vi "locate tag.vi"(8 "error in":errorcluster, 10 "name":string, 11 "data dictionary in":refnum<class "data bus dictionary.lvclass">) -> (0 "error out":errorcluster, 1 "data type":T1, 2 "index":i32, 3 "data dictionary out":refnum<class "data bus dictionary.lvclass">)   [LabVIEW 2013, in "data bus dictionary.lvclass"]
doc: "Locates a tag in the data dictionary and returns its index within the data table."
uses:
  data bus dictionary.lvclass
  tag/Data Type.ctl
  data bus dictionary.lvclass/data bus dictionary.ctl
  dictionary lookup value.ctl
  tag/data bus tag description.lvclass
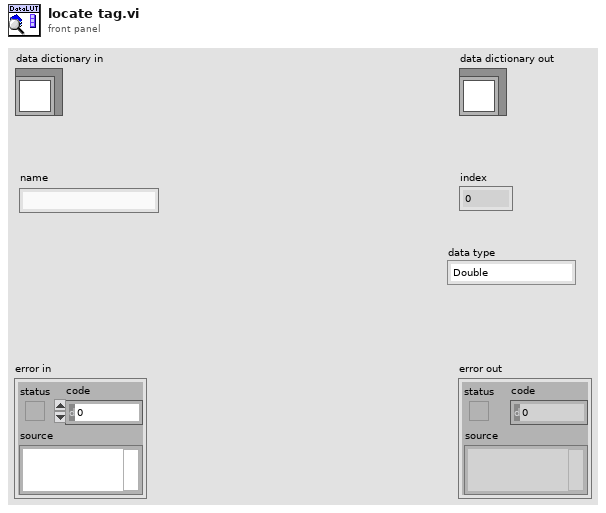
[diagram p1: front panel]
types:
  T1 = typedef "data bus tag description.lvclass/Data Type.ctl" = enum16{"Double", "I64", "Boolean", "Array of Double", "Array of I64", "Variant"}
  T2 = typedef "data bus dictionary.lvclass/dictionary lookup value.ctl" = cluster{"data type":T1, "index":i32}
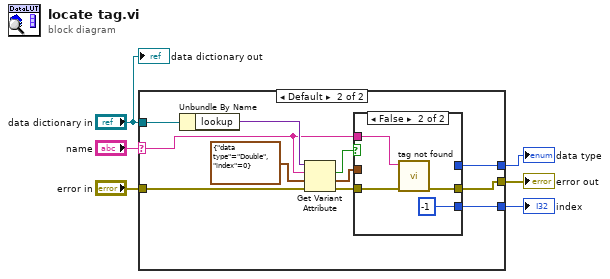
[diagram p0: block diagram]
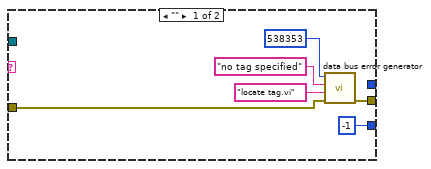
[diagram p2: hidden frame]
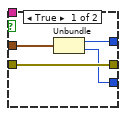
[diagram p3: hidden frame]
diagram:
  n1 = case shown="Default" "name" {
    selector: "name" -> [_ w18]
    tunnel: "data dictionary in" -> [_ w21]
    tunnel: "error in" -> [w10 w23]
    tunnel: [w11 w22] -> w4
    tunnel: [-1 ("data index") w13] -> w3
    tunnel: [_ w14] -> w1
    frame "" {
      n2 = call "data bus error generator.vi"("error in"=w10, "source"="locate tag.vi", "append error message"="no tag specified", "error code (0)"=538353) -> ("error out"=w11:errorcluster)  [unwired: 5 in]
    }
    frame Default {
      n3 = Unbundle By Name(w21) -> ("lookup"=w19:variant)
      n4 = Get Variant Attribute(Variant=w19, name=w18, default value (empty Variant)=T2 {"data type"=enum."Double", "index"=0} ("dictionary lookup"), error in=w23) -> (found=w16:bool, value=w15:T2, error out=w20:errorcluster)  [unwired: 1 out]
      n5 = case shown="False" w16 {
        tunnel: w20 -> [w27 w31]
        tunnel: [w27 w30] -> w22
        tunnel: w18 -> [_ w29]
        tunnel: w15 -> [w26 _]
        tunnel: [w25 _] -> w14
        tunnel: [w24 -1 ("index")] -> w13
        frame True {
          n6 = Unbundle(w26) -> ("data type"=w25:T1, "index"=w24:i32)
        }
        frame False {
          n7 = call "tag not found.vi"("error in"=w31, "name"=w29) -> ("error out"=w30:errorcluster)  [unwired: 9 in]
        }
      }
    }
  }
  "error out" <- w4
  "data type" <- w1
  "index" <- w3
  "data dictionary out" <- "data dictionary in"
